vi "FisherPaykel Spin PID.vi"(7 "Debug":bool, 8 "Error In":errorcluster, 10 "Spin PID":T1={"Kp"=1.84, "Ki"=0.03, "Kd"=0.0, "Kc"=0.06} {"Kc" min=0.0 max=1.0; "Kd" min=0.0 max=1.0; "Ki" min=0.0 max=1.0; "Kp" min=0.0 max=16.0}, 11 "VISA Refnum in":refnum<visa-resource-name>) -> (0 "Error Out":errorcluster, 3 "VISA Refnum out":refnum<visa-resource-name>)   [LabVIEW 2016]
uses:
  Type Definitions/Fisher Paykel Spin PID.ctl
panel:
  out "Send Command":string
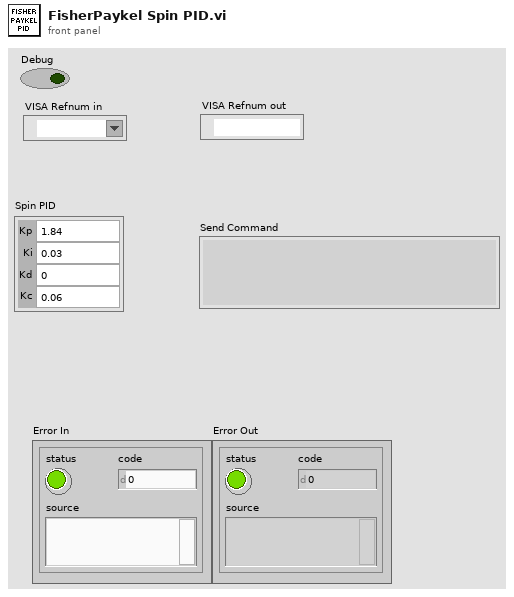
[diagram p1: front panel]
types:
  T1 = typedef "Fisher Paykel Spin PID.ctl" = cluster{"Kp":dbl, "Ki":dbl, "Kd":dbl, "Kc":dbl}
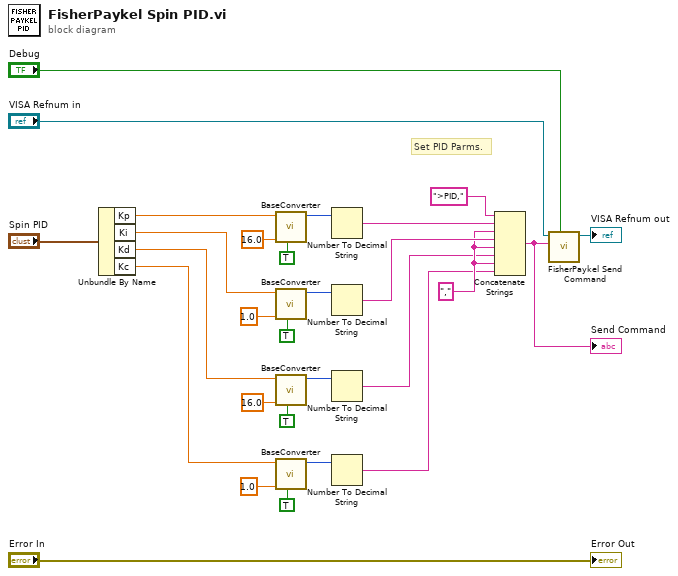
[diagram p0: block diagram]
diagram:
  w12 = "," ("string")
  # "Set PID Parms."
  n1 = Unbundle By Name("Spin PID") -> ("Kp"=w25:dbl, "Ki"=w24:dbl, "Kd"=w23:dbl, "Kc"=w22:dbl)
  n2 = call "BaseConverter.vi"("Action"=TRUE, "Base"=16.0, "Input"=w25) -> ("Output"=w17:i16)  [unwired: 8 in]
  n3 = call "BaseConverter.vi"("Action"=TRUE, "Base"=1.0, "Input"=w24) -> ("Output"=w16:i16)  [unwired: 8 in]
  n4 = call "BaseConverter.vi"("Action"=TRUE, "Base"=16.0, "Input"=w23) -> ("Output"=w19:i16)  [unwired: 8 in]
  n5 = call "BaseConverter.vi"("Action"=TRUE, "Base"=1.0, "Input"=w22) -> ("Output"=w18:i16)  [unwired: 8 in]
  n6 = Number To Decimal String(number=w17) -> (decimal integer string=w14:string)  [unwired: 1 in]
  n7 = Number To Decimal String(number=w16) -> (decimal integer string=w13:string)  [unwired: 1 in]
  n8 = Number To Decimal String(number=w19) -> (decimal integer string=w11:string)  [unwired: 1 in]
  n9 = Number To Decimal String(number=w18) -> (decimal integer string=w10:string)  [unwired: 1 in]
  n10 = Concatenate Strings(">PID,", w14, w12, w13, w12, w11, w12, w10) -> (w27:string)
  "Send Command" <- w27
  n11 = call "FisherPaykel Send Command.vi"("Debug"="Debug", "Send Command"=w27, "VISA Refnum in"="VISA Refnum in") -> ("VISA Refnum out"=→"VISA Refnum out":refnum<visa-resource-name>)  [unwired: 6 in, 2 out]
  "Error Out" <- "Error In"
